vi "Write Notifiers.vi"(10 "Notifiers":T1, 11 "IED Test in":refnum<class "IED Test.lvclass">) -> (3 "IED Test out":refnum<class "IED Test.lvclass">)   [LabVIEW 2018, in "IED Test Framework.lvlib" / "IED Test.lvclass"]
uses:
  IED Test.lvclass
  EMS Core/EMS/Controls/Notifiers.ctl
  IED Test.lvclass/IED Test.ctl
  EMS Core/EMS/EMS.lvclass
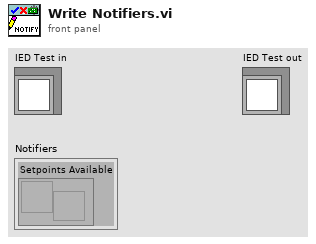
[diagram p1: front panel]
types:
  T1 = typedef "EMS Core.lvlib/EMS.lvclass/Notifiers.ctl" = cluster{"Setpoints Available":refnum<notifier>}
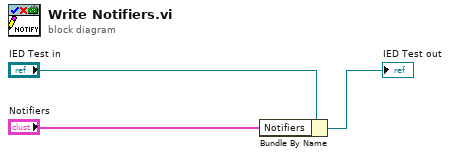
[diagram p0: block diagram]
diagram:
  n1 = Bundle By Name(cluster="IED Test in", "Notifiers"="Notifiers") -> (→"IED Test out":refnum<class "IED Test.lvclass">)
